vi "Get Version.vi"(8 "error in":errorcluster, 11 "RDMA Configurations in":refnum<class "RDMA Configurations.lvclass">) -> (0 "error out":errorcluster, 2 "version":T1, 3 "RDMA Configurations out":refnum<class "RDMA Configurations.lvclass">)   [LabVIEW 2020, in "RDMA.lvlib" / "RDMA Configurations.lvclass"]
uses:
  RDMA Configurations.lvclass
  DSF Core.lvlibp/Typedefs/DSF Version Info.ctl
  DSF Core.lvlibp
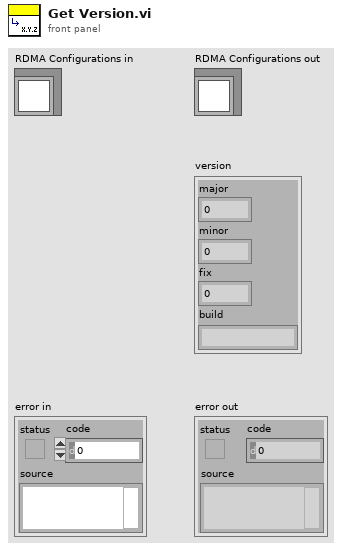
[diagram p1: front panel]
types:
  T1 = typedef "DSF Core.lvlibp/DSF Version Info.ctl" = cluster{"major":u32, "minor":u32, "fix":u32, "build":string}
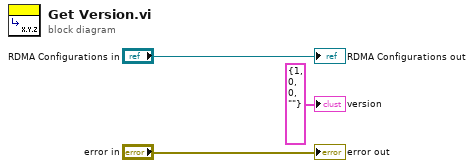
[diagram p0: block diagram]
diagram:
  "error out" <- "error in"
  "RDMA Configurations out" <- "RDMA Configurations in"
  "version" <- T1 {"major"=1, "minor"=0, "fix"=0, "build"=""} ("version")
